vi "TestExec.Example Station Module.vi"(11 "Module Config":T1={"Name"="CircleTest", "Parent Q"=refnum, "Is Child?"=FALSE, "Index"=0, "Dirs"={"Root"=path "", "Config"=path "C:/ATE/Config", "Logs"=path "C:/ATE/Logs", "Reports"=path "C:/ATE/Reports", "App Data"=path "C:/ProgramData/MAIN"}, "Simulate"=FALSE, "SimCtrl"=refnum}) -> ()   [LabVIEW 2018]
uses:
  <vilib>/KATE/Queues/Queue Utils.lvlib
  <vilib>/KATE/Module/Module Utils.lvlib
  <vilib>/KATE/Module/Window/Window.Task, Action.ctl
  <vilib>/KATE/Event Log/Event Log.lvlib
  <vilib>/KATE/Scheduler/Scheduler.lvlib
  <vilib>/KATE/Menu/Menu Utils.lvlib
  <vilib>/KATE/Config/Config Utils.lvlib
  Base Station/Circle Test/Controls & TypeDefs/CircleTest.Config, Track Object Table.ctl
  Common/Utils/Logging/Log Level.ctl
  Common/Utils/Logging/Log Params.ctl
  <vilib>/KATE/Config/Stored Controls/Class.SaveCtrls.lvclass
  <vilib>/KATE/Queues/Q.Element.ctl
  <vilib>/KATE/Module/Module Config.ctl
  <vilib>/KATE/Module/Module.Working Dirs.ctl
  <vilib>/KATE/Module/Module.SW Version Info.ctl
panel:
  in  "Main Tab":enum32{"Operate", "Maint"}(tab)
  out "Simulate Indication":string="Simulating Instruments"
  in  "Data Tab":enum32{"Test Control", "Config"}(tab)
  out "Status":string
  in  "Logging Level":i32
  out "Rev":string="v1.0.0"
  in  "Leave Maint":bool
  in  "SW Rev":T3={"AppName"="Circle Test", "Company"="Valve", "Version"="1.0", "Description"="", "PN"=""}
  # "Title"
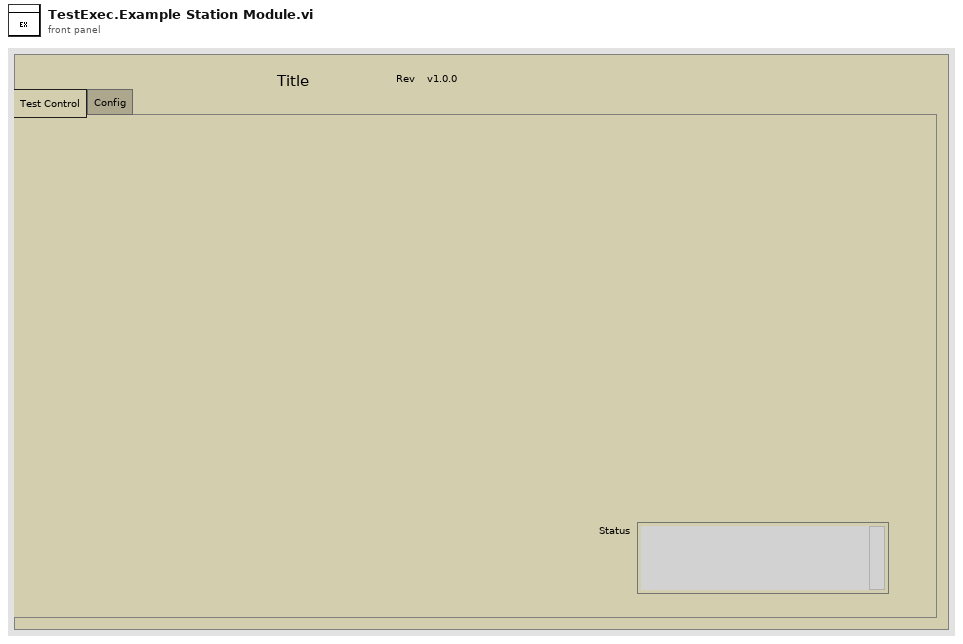
[diagram p1: front panel]
types:
  T1 = typedef "KATE_Lib.lvlib/Module Utils.lvlib/Module Config.ctl" = cluster{"Name":string, "Parent Q":refnum<queue>, "Is Child?":bool, "Index":i32, "Dirs":T2, "Simulate":bool, "SimCtrl":refnum<vi>}
  T2 = typedef "KATE_Lib.lvlib/Module Utils.lvlib/Module.Working Dirs.ctl" = cluster{"Root":path, "Config":path, "Logs":path, "Reports":path, "App Data":path}
  T3 = typedef "KATE_Lib.lvlib/Module Utils.lvlib/Module.SW Version Info.ctl" = cluster{"AppName":string, "Company":string, "Version":string, "Description":string, "PN":string}
  T4 = typedef "KATE_Lib.lvlib/Module Utils.lvlib/Module Sys Info.ctl" = cluster{"Main Q":refnum<queue>, "Exe":bool, "SW Rev":T3, "Self Ref":refnum<vi>, "Main Tab":refnum<vi>, "Pane":refnum<vi>, "Stop":cluster{"Ref":refnum<event-registration>, "Event":refnum<user-event>}, "Cfg":T1, "Services":cluster{"Name":string, "vi ref":refnum<vi>}[], "Menu Ref":refnum<k9>, "CtrlStates":refnum<class "Class.SaveCtrls.lvclass">, "Docs":cluster{"Tags":string[], "Paths":path[]}, "Log":refnum<class "Event Notification.lvclass">, "Test Controls":refnum<vi>[], "Child Modules":cluster{"Name":string, "vi ref":refnum<vi>}[], "SW Items":string[][], "AppData":refnum<class "Class.AppData.lvclass">}
  T5 = enum8{"Enabled", "Disabled", "Disabled and Grayed Out"}
  T6 = typedef "Log Params.ctl" = cluster{"Log Level":T7, "StatusTxtBoxRef":refnum<vi>, "AppID":string, "Is Child?":bool, "Parent Q":refnum<queue>}
  T7 = typedef "Log Level.ctl" = enum16{"Normal", "Verbose", "Debug0", "Debug1", "Debug2"}
  T8 = typedef "CircleTest.Config, Track Object Table.ctl" = cluster{"SNs":string[], "Enable":bool[]}
  T9 = cluster{"Child Modules":cluster{"VI Ref":refnum<vi>, "Name":string}[]}
  T10 = cluster{"Lnch":bool, "Track Obj Config":T8, "Log":T6, "XX":string, "App":cluster{"Child Modules":cluster{"VI Ref":refnum<vi>, "Name":string}[]}}
  T11 = typedef "KATE_Lib.lvlib/Module Utils.lvlib/Window.Task, Action.ctl" = enum16{"Resize()", "Show Panel(Bool)", "Show Scroll Bars(Bool)", "Dock to SubPanel(SubPanel Ref)", "Undock from SubPanel()", "Return to SubPanel()", "Go To Maint Tab()", "Show Maint Tab(Bool)", "Open Block Diagram()"}
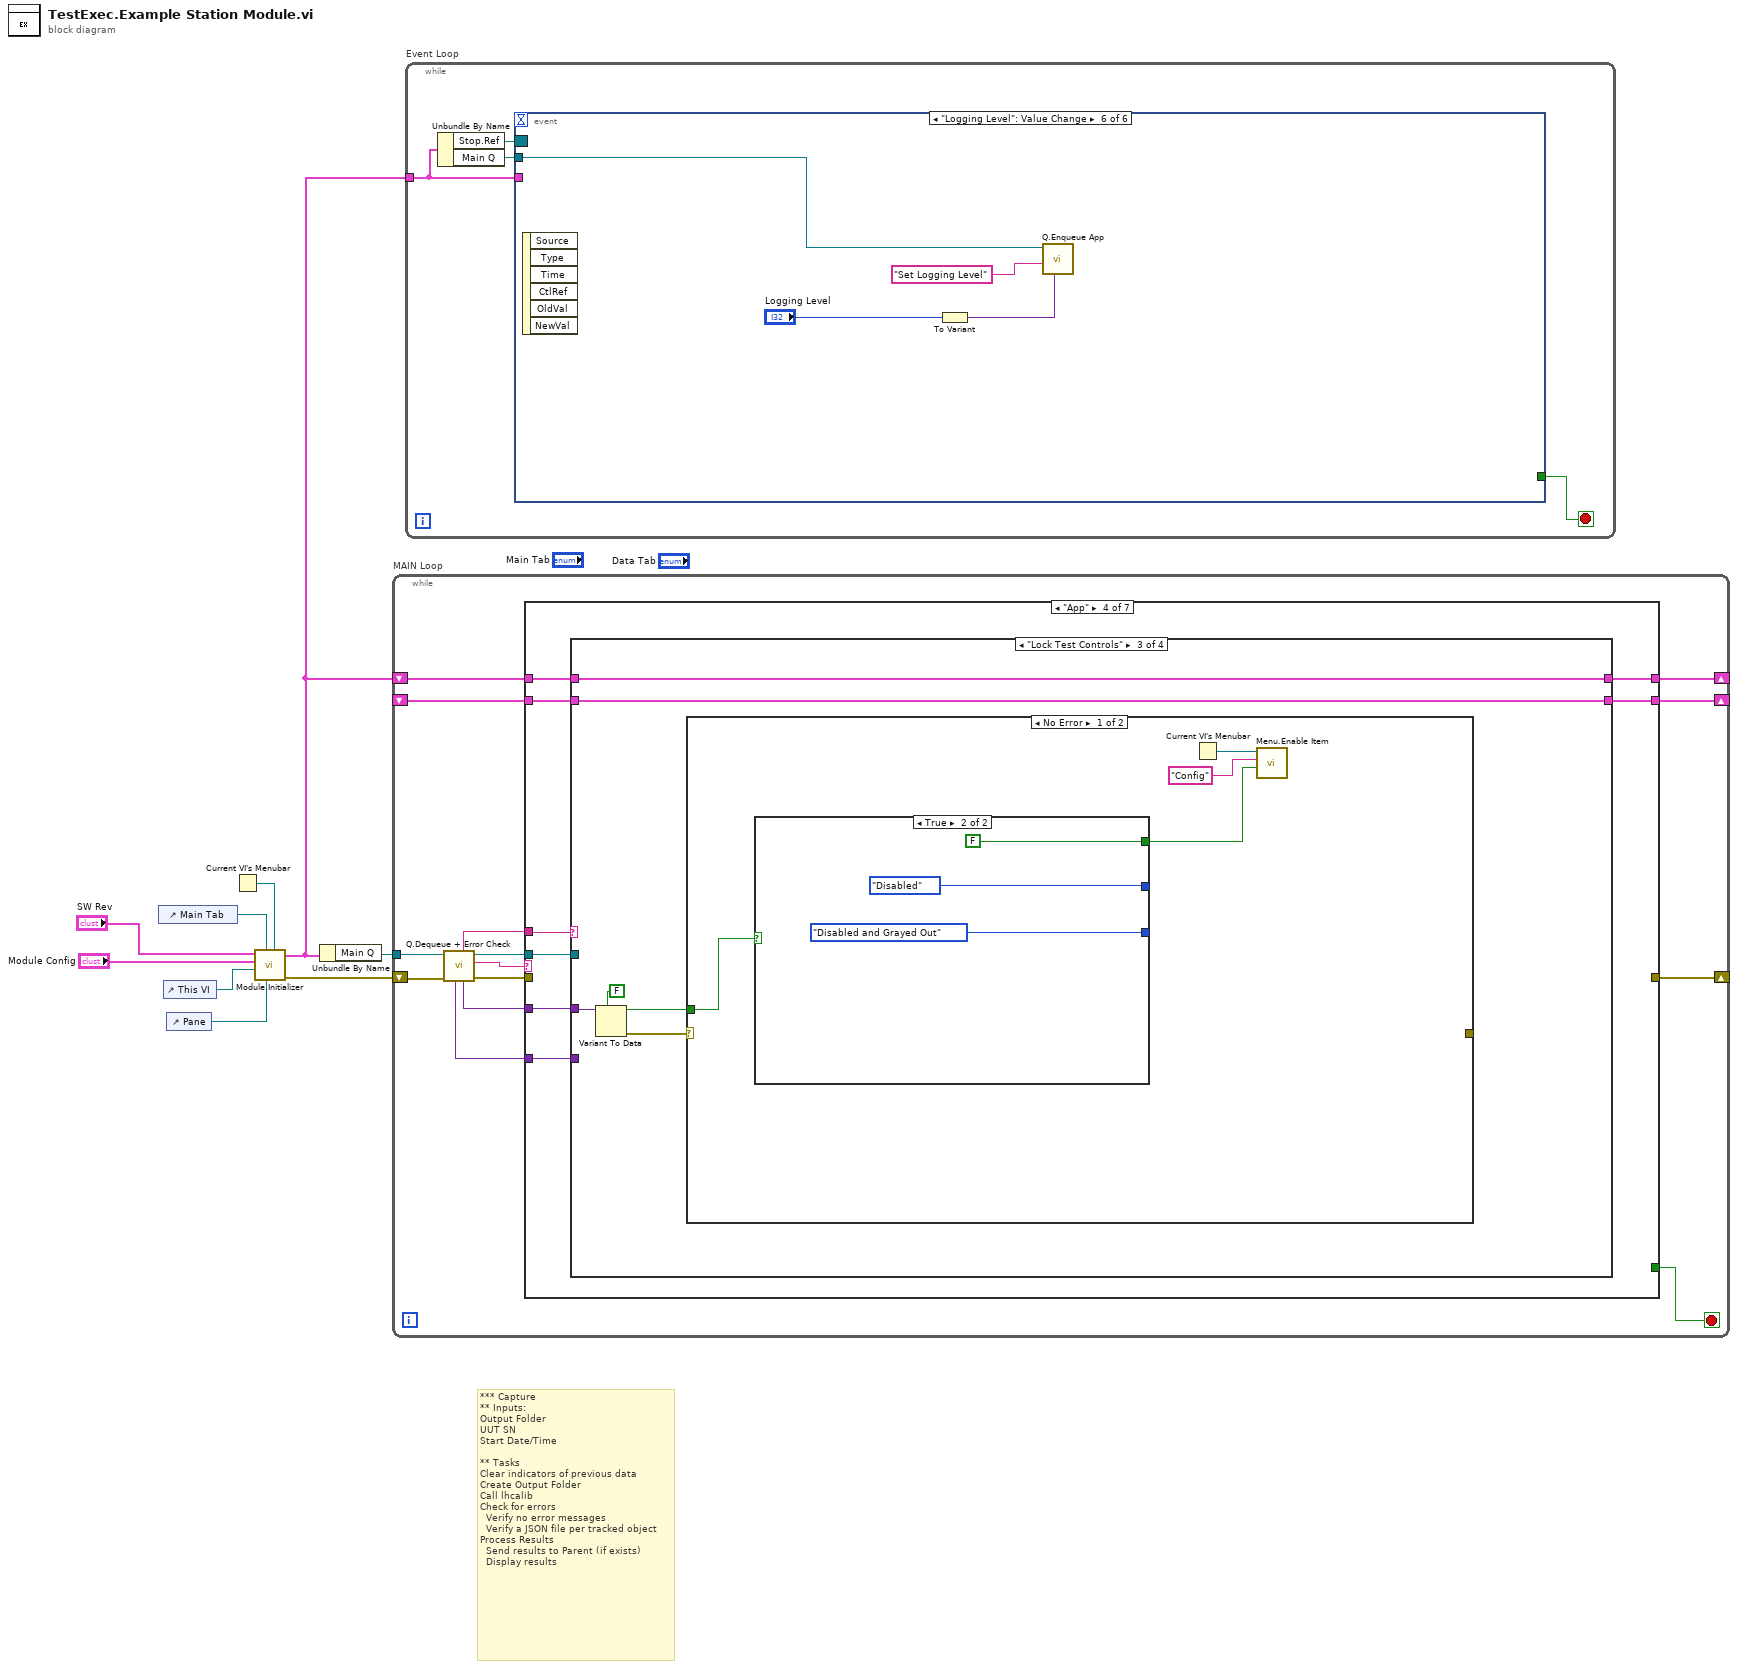
[diagram p0: block diagram]
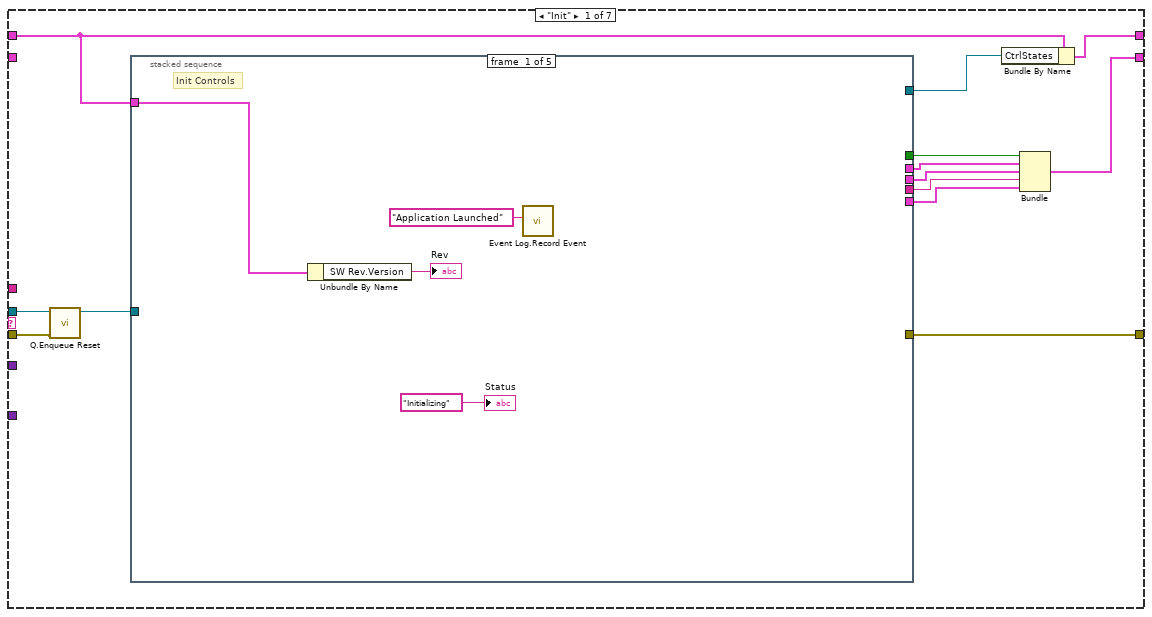
[diagram p2: hidden frame]
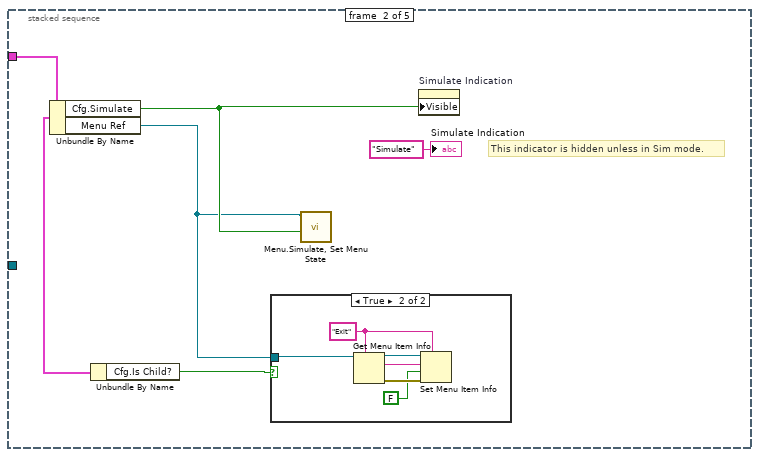
[diagram p3: hidden frame]
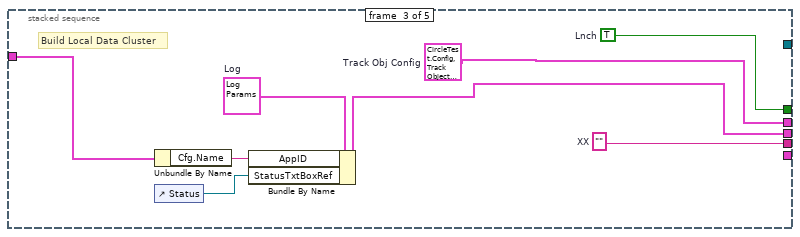
[diagram p5: hidden frame]
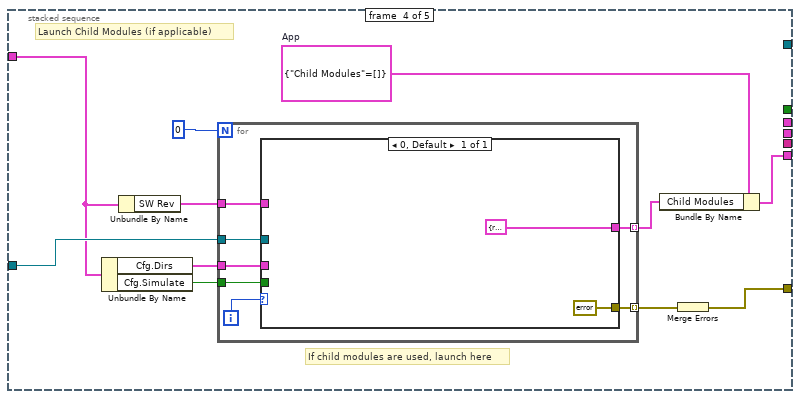
[diagram p6: hidden frame]
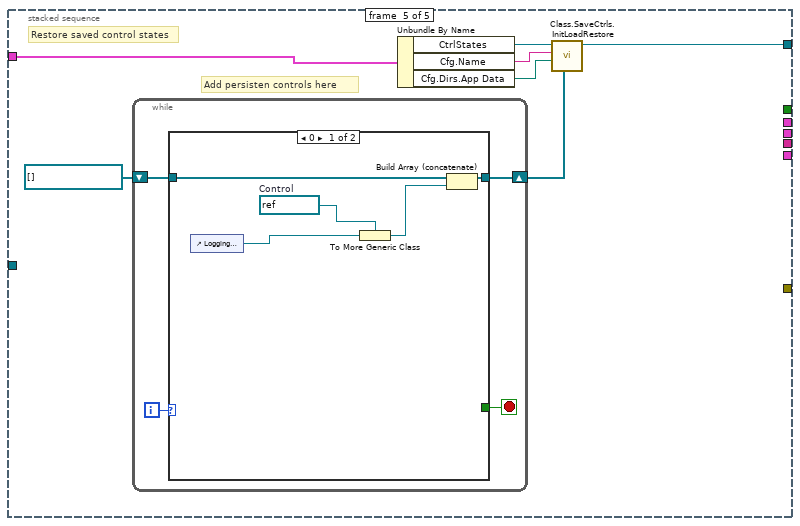
[diagram p7: hidden frame]
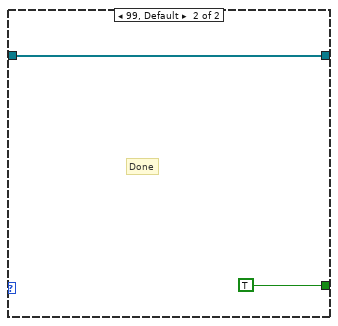
[diagram p8: hidden frame]
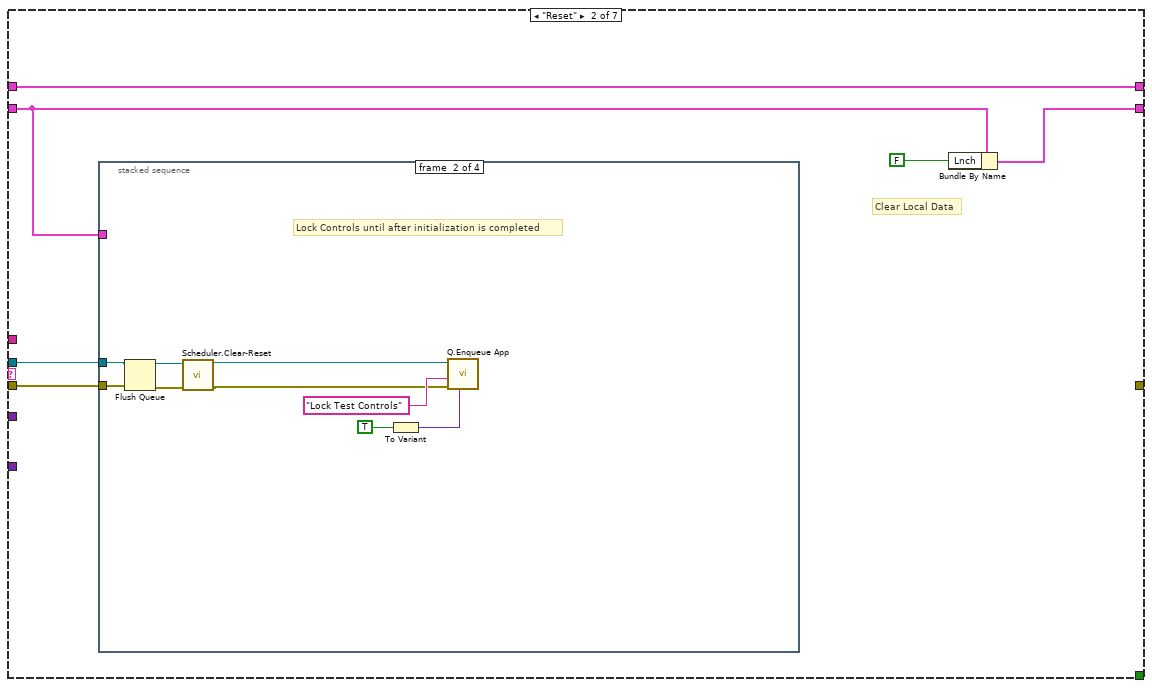
[diagram p9: hidden frame]
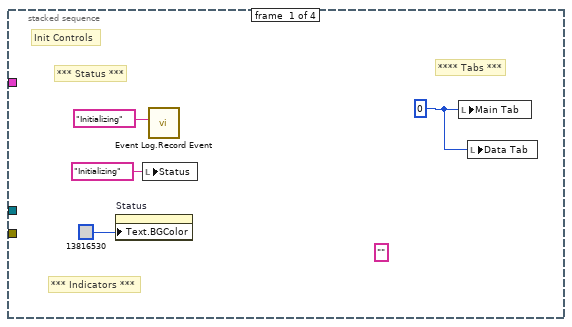
[diagram p10: hidden frame]
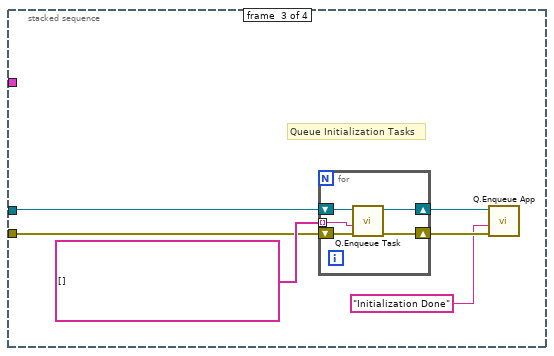
[diagram p11: hidden frame]
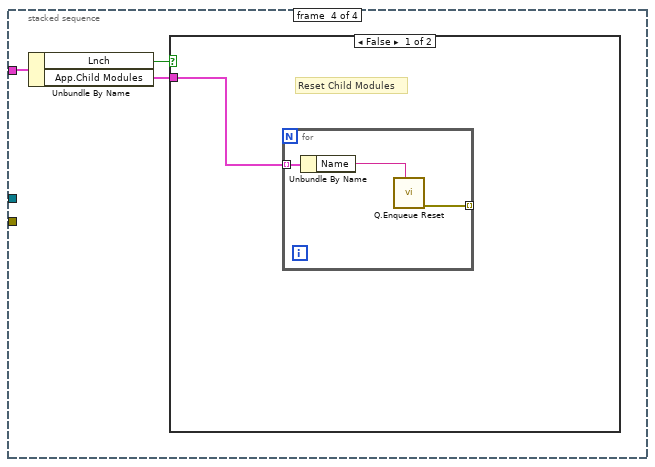
[diagram p12: hidden frame]
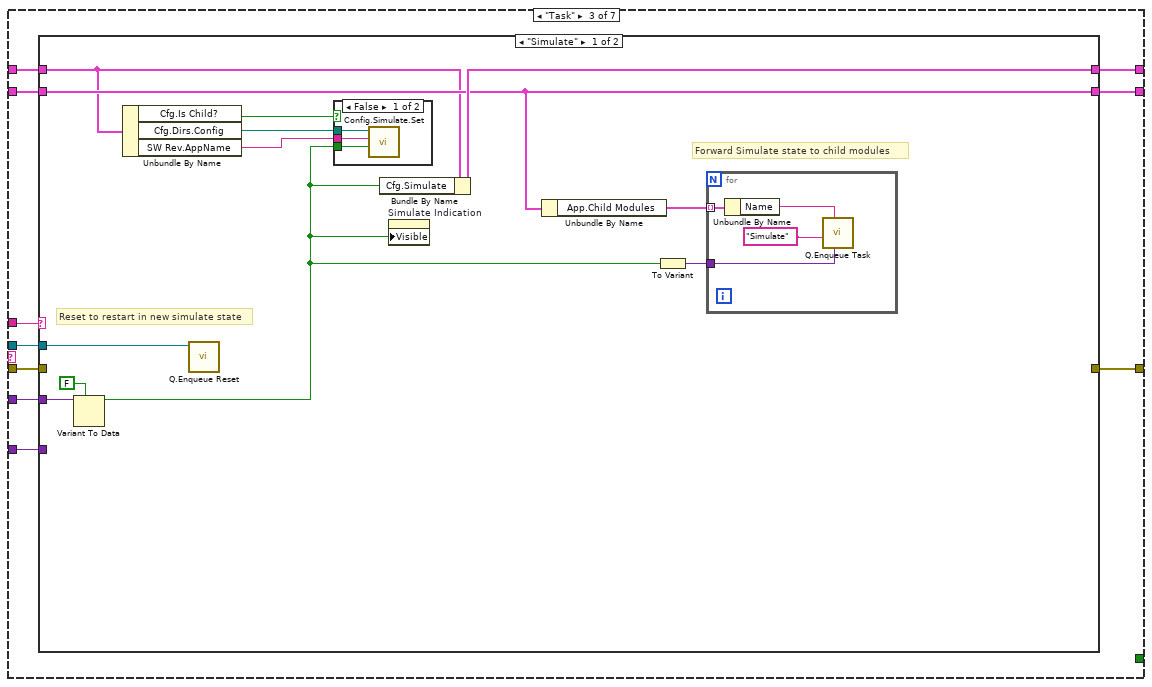
[diagram p14: hidden frame]
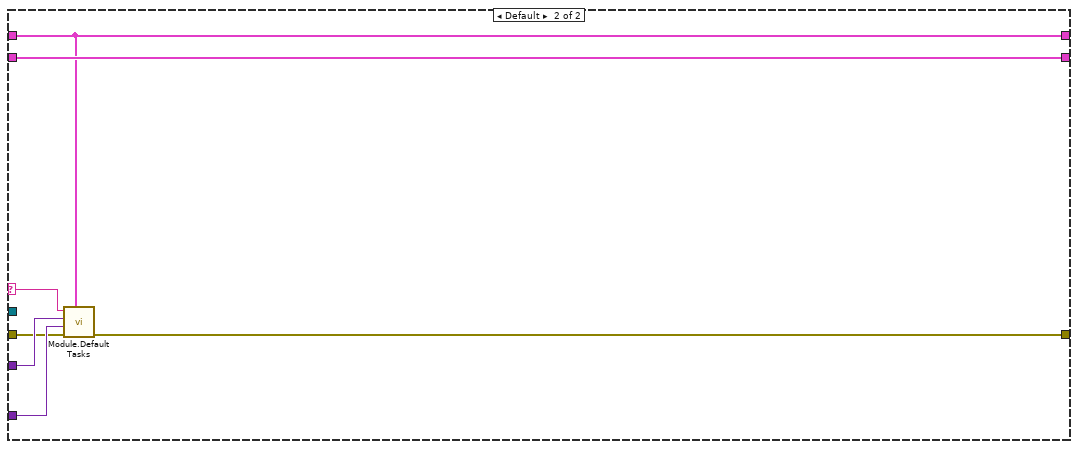
[diagram p16: hidden frame]
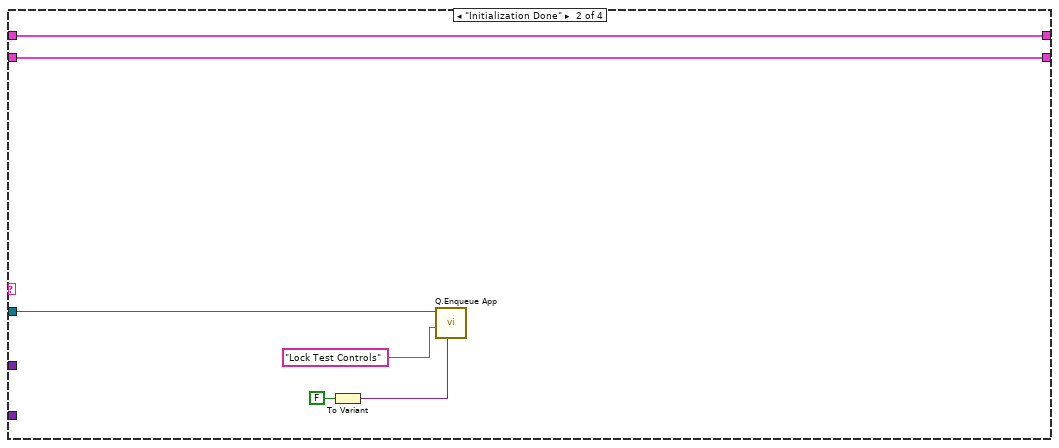
[diagram p18: hidden frame]
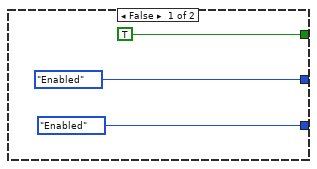
[diagram p19: hidden frame]
diagram:
  # "*** Capture\n** Inputs:\nOutput Folder\nUUT SN\nStart Date/Time\n\n** Tasks \nClear indicators of previous data\nCreate Output Folder\nCall lhcalib\nCheck for errors\n  Verify no error messages\n  Verify a JSON file per tracked object\nProcess Results\n  Send results to Parent (if exists)\n  Display results"
  n1 = control-ref of="Main Tab"() -> (w7:refnum<vi>)
  n2 = control-ref of="This VI"() -> (w6:refnum<vi>)
  n3 = control-ref of="Pane"() -> (w5:refnum<vi>)
  n4 = Current VI's Menubar() -> (w3:refnum<k9>)
  n5 = call <vilib>:"Module.Initializer.vi"("Menu Ref"=w3, "Pane"=w5, "Main Tab"=w7, "Self Ref"=w6, "Module Config"="Module Config", "SW Rev"="SW Rev") -> ("error out"=w9:errorcluster, "Sys"=w4:T4)  [unwired: 4 in]
  n6 = Unbundle By Name(w4) -> ("Main Q"=w8:refnum<queue>)
  n7 = while "MAIN Loop" {
    shift-right: [w19] -> _
    shift-left: w9 -> [w17]
    shift-right: [w20] -> _
    shift-left: _ -> [w23]
    shift-right: [w21] -> _
    shift-left: w4 -> [w22]
    tunnel: w8 -> [w16]
    stop <- w11 stop-if-true
    n8 = call <vilib>:"Q.Dequeue + Error Check.vi"("Error In"=w17, "Q In"=w16) -> ("error out"=w18:errorcluster, "Cmd"=w15:string, "Q Out"=w14:refnum<queue>, "Data1"=w13:variant, "Sub"=w10:string, "Data2"=w12:variant)  [unwired: 4 in]
    n9 = case shown="\"App\"" w15 {
      selector: w15 -> [_ _ _ _ _ w230 _]
      tunnel: w23 -> [_ w99 w143 w173 w220 w232 w259]
      tunnel: w22 -> [w29 w102 w144 w174 w221 w233 w260]
      tunnel: [w30 w102 w142 w172 w219 w233 w260] -> w21
      tunnel: [w34 w103 w141 w171 w218 w232 w259] -> w20
      tunnel: [w26 _ w135 _ w213 w231 w262] -> w19
      tunnel: w18 -> [w35 w100 w137 _ w214 w228 _]
      tunnel: w14 -> [w36 w101 w138 w177 w215 w226 _]
      tunnel: w13 -> [_ _ w139 w176 w216 w229 _]
      tunnel: w12 -> [_ _ w136 w175 w212 _ _]
      tunnel: w10 -> [_ _ w140 w178 w217 w227 _]
      tunnel: [_ _ _ _ _ _ TRUE] -> w11
      frame "Init" {
        n10 = call <vilib>:"Q.Enqueue Reset.vi"("Error In"=w35, "Q In"=w36) -> ("Q Out"=w27:refnum<queue>)  [unwired: 8 in, 1 out]
        n11 = stacked-sequence {
          tunnel: [_ _ w58 _ _] -> w33
          tunnel: [_ _ w56 _ _] -> w32
          tunnel: [_ _ w52 _ _] -> w31
          tunnel: w29 -> [w38 w42 w55 w63 w81]
          tunnel: [_ _ _ _ w80] -> w28
          tunnel: [_ _ _ w69 _] -> w24
          tunnel: w27 -> [_ _ _ w64 _]
          tunnel: [_ _ _ w60 _] -> w26
          tunnel: [_ _ w59 _ _] -> w25
          frame #0 {
            # "Init Controls"
            n12 = Unbundle By Name(w38) -> ("SW Rev.Version"=→"Rev":string)
            n13 = call <vilib>:"Event Log.Record Event.vi"("Message"="Application Launched") -> ()  [unwired: 10 in, 1 out]
            "Status" <- "Initializing" ("Status")
          }
          frame #1 {
            # "This indicator is hidden unless in Sim mode."
            n14 = Unbundle By Name(w42) -> ("Cfg.Simulate"=w44:bool, "Menu Ref"=w41:refnum<k9>)
            n15 = Unbundle By Name(w42) -> ("Cfg.Is Child?"=w43:bool)
            n16 = case shown="True" w43 {
              tunnel: w41 -> [_ w47]
              frame False {
              }
              frame True {
                w49 = "Exit"
                n17 = Get Menu Item Info(7:w49, 11:w47) -> (0:w48:errorcluster, 2:w50:string, 3:w51:refnum<k9>)  [unwired: 1 in, 4 out]
                n18 = Set Menu Item Info(7:w49, 8:w48, 9:FALSE ("enabled"), 10:w50, 11:w51) -> ()  [unwired: 2 in, 2 out]
              }
            }
            n19 = call <vilib>:"Menu.Simulate, Set Menu State.vi"("Sim Enable"=w44, "Menu Ref"=w41) -> ()  [unwired: 8 in, 2 out]
            n20 = property on="Simulate Indication" class="Str"("Visible"=w44) -> ()  [unwired: 2 in, 2 out]
            "Simulate Indication" <- "Simulate" ("Simulate Indication")
          }
          frame #2 {
            w52 = ""  # XX
            w57 = T6 {"Log Level"=enum."Normal", "StatusTxtBoxRef"=refnum, "AppID"="", "Is Child?"=FALSE, "Parent Q"=refnum}  # Log
            w58 = T8 {"SNs"=["", "", "", "", "", "", "", "", "", "", "", "", "", ""], "Enable"=[TRUE, TRUE, TRUE, TRUE, TRUE, TRUE, TRUE, TRUE, TRUE, TRUE, TRUE, TRUE, TRUE, TRUE]}  # Track Obj Config
            w59 = TRUE  # Lnch
            # "Build Local Data Cluster"
            n21 = Unbundle By Name(w55) -> ("Cfg.Name"=w54:string)
            n22 = control-ref of="Status"() -> (w53:refnum<vi>)
            n23 = Bundle By Name(cluster=w57, "AppID"=w54, "StatusTxtBoxRef"=w53) -> (w56:T6)
          }
          frame #3 {
            w70 = T9 {"Child Modules"=[]}  # App
            # "If child modules are used, launch here"
            # "Launch Child Modules (if applicable)"
            n24 = Unbundle By Name(w63) -> ("Cfg.Dirs"=w66:T2, "Cfg.Simulate"=w65:bool)
            n25 = Unbundle By Name(w63) -> ("SW Rev"=w68:T3)
            n26 = for {
              N: 0 -> [_]
              tunnel: w68 -> [w77]
              tunnel: [w72] -> w62 mode=indexing
              tunnel: w64 -> [w75]
              tunnel: w66 -> [w74]
              tunnel: w65 -> [w73]
              tunnel: [w71] -> w61 mode=indexing
              i -> [w76]
              n27 = case shown="0, Default" w76 {
                tunnel: w77 -> [_]
                tunnel: w75 -> [_]
                tunnel: w74 -> [_]
                tunnel: w73 -> [_]
                tunnel: [cluster{"VI Ref":refnum<vi>, "Name":string} {"VI Ref"=refnum, "Name"=""} ("output cluster")] -> w72
                tunnel: [errorcluster {"status"=FALSE, "code"=0, "source"=""} ("error constant")] -> w71
                frame 0, Default {
                }
              }
            }
            n28 = Bundle By Name(cluster=w70, "Child Modules"=w62) -> (w69:T9)
            n29 = Merge Errors(w61) -> (w60:errorcluster)
          }
          frame #4 {
            # "Add persisten controls here"
            # "Restore saved control states"
            n30 = while {
              shift-right: [w88] -> w82
              shift-left: refnum<vi>[] [] -> [w89]
              i -> [w90]
              stop <- w87 stop-if-true
              n31 = case shown="0" w90 {
                tunnel: w89 -> [w94 w97]
                tunnel: [w95 w97] -> w88
                tunnel: [_ TRUE] -> w87
                frame 0 {
                  w92 = refnum<vi> refnum  # Control
                  n32 = control-ref of="Logging Level"() -> (w91:refnum<vi>)
                  n33 = To More Generic Class(target class=w92, reference=w91) -> (generic class reference=w93:refnum<vi>)
                  n34 = Build Array (concatenate)(w94, w93) -> (w95:refnum<vi>[])
                }
                frame 99, Default {
                  # "Done"
                }
              }
            }
            n35 = Unbundle By Name(w81) -> ("CtrlStates"=w83:refnum<class "Class.SaveCtrls.lvclass">, "Cfg.Name"=w85:string, "Cfg.Dirs.App Data"=w84:path)
            n36 = call-dynamic "Class.SaveCtrls.InitLoadRestore.vi"("Ctrl Array"=w82, "Module Data Dir"=w84, "Module Name"=w85, "CtrlStates In"=w83) -> ("CtrlStates"=w80:refnum<class "Class.SaveCtrls.lvclass">)  [unwired: 6 in, 1 out]
          }
        }
        n37 = Bundle By Name(cluster=w29, "CtrlStates"=w28) -> (w30:T4)
        n38 = Bundle("Lnch"=w25, "Track Obj Config"=w33, "Log"=w32, "XX"=w31, "App"=w24) -> (w34:T10)  [unwired: 1 in]
      }
      frame "Reset" {
        # "Clear Local Data"
        n39 = stacked-sequence {
          tunnel: w101 -> [_ w109 w117 _]
          tunnel: w100 -> [_ w108 w121 _]
          tunnel: w99 -> [_ _ _ w130]
          frame #0 {
            (unwired) "" ("Log")
            w104 = 0
            # "*** Indicators ***"
            # "**** Tabs ***"
            # "*** Status ***"
            # "Init Controls"
            n40 = property on="Status" class="Str"("Text.BGColor"=u32 13816530) -> ()  [unwired: 2 in, 2 out]
            n41 = local write "Status"("Initializing" ("Status")) -> ()
            n42 = call <vilib>:"Event Log.Record Event.vi"("Message"="Initializing") -> ()  [unwired: 10 in, 1 out]
            n43 = local write "Main Tab"(w104) -> ()
            n44 = local write "Data Tab"(w104) -> ()
          }
          frame #1 {
            # "Lock Controls until after initialization is completed"
            n45 = Flush Queue(queue=w109, error in (no error)=w108) -> (queue out=w110:refnum<queue>, error out=w113:errorcluster)  [unwired: 1 out]
            n46 = call <vilib>:"Scheduler.Clear-Reset.vi"("error in"=w113, "Q In"=w110) -> ("error out"=w111:errorcluster, "Q Out"=w112:refnum<queue>)  [unwired: 8 in]
            n47 = To Variant(anything=TRUE) -> (Variant=w115:variant)
            n48 = call <vilib>:"Q.Enqueue App.vi"("Data1"=w115, "Error In"=w111, "Task Name"="Lock Test Controls", "Q In"=w112) -> ()  [unwired: 6 in, 2 out]
          }
          frame #2 {
            # "Queue Initialization Tasks"
            n49 = for {
              shift-right: [w125] -> w119
              shift-left: w121 -> [w126]
              tunnel: string[] [] -> [w123] mode=indexing
              shift-right: [w124] -> w120
              shift-left: w117 -> [w127]
              n50 = call <vilib>:"Q.Enqueue Task.vi"("Error In"=w126, "Task Name"=w123, "Q In"=w127) -> ("error out"=w125:errorcluster, "Q Out"=w124:refnum<queue>)  [unwired: 7 in]
            }
            n51 = call <vilib>:"Q.Enqueue App.vi"("Error In"=w119, "Task Name"="Initialization Done", "Q In"=w120) -> ()  [unwired: 7 in, 2 out]
          }
          frame #3 {
            n52 = Unbundle By Name(w130) -> ("Lnch"=w129:bool, "App.Child Modules"=w128:cluster{"VI Ref":refnum<vi>, "Name":string}[])
            n53 = case shown="False" w129 {
              tunnel: w128 -> [w131 _]
              frame False {
                # "Reset Child Modules"
                n54 = for {
                  tunnel: w131 -> [w134] mode=indexing
                  tunnel: [w132] -> _ mode=indexing
                  n55 = Unbundle By Name(w134) -> ("Name"=w133:string)
                  n56 = call <vilib>:"Q.Enqueue Reset.vi"("Q Name"=w133) -> ("error out"=w132:errorcluster)  [unwired: 9 in, 1 out]
                }
              }
              frame True {
                # "Do not reset at launch.\nThey are already reset"
              }
            }
          }
        }
        n57 = Bundle By Name(cluster=w99, "Lnch"=FALSE ("Test.Running")) -> (w103:T10)
      }
      frame "Task" {
        n58 = case shown="\"Simulate\"" w140 {
          selector: w140 -> [_ w168]
          tunnel: w144 -> [w149 w169]
          tunnel: w143 -> [w153 w170]
          tunnel: [w154 w169] -> w142
          tunnel: [w153 w170] -> w141
          tunnel: w139 -> [w156 w167]
          tunnel: w138 -> [w150 _]
          tunnel: w137 -> [_ w165]
          tunnel: w136 -> [_ w166]
          tunnel: [_ w164] -> w135
          frame "Simulate" {
            # "Reset to restart in new simulate state"
            # "Forward Simulate state to child modules"
            n59 = Variant To Data(type=FALSE, Variant=w156) -> (data=w146:bool)  [unwired: 1 in, 1 out]
            n60 = Unbundle By Name(w149) -> ("Cfg.Is Child?"=w145:bool, "Cfg.Dirs.Config"=w148:path, "SW Rev.AppName"=w147:string)
            n61 = call <vilib>:"Q.Enqueue Reset.vi"("Q In"=w150) -> ()  [unwired: 9 in, 2 out]
            n62 = case shown="False" w145 {
              tunnel: w148 -> [w159 _]
              tunnel: w147 -> [w158 _]
              tunnel: w146 -> [w157 _]
              frame False {
                n63 = call <vilib>:"Config.Simulate.Set.vi"("Simulate"=w157, 10:w158, "Config Folder"=w159) -> ()  [unwired: 8 in, 1 out]
              }
              frame True {
              }
            }
            n64 = Bundle By Name(cluster=w149, "Cfg.Simulate"=w146) -> (w154:T4)
            n65 = property on="Simulate Indication" class="Str"("Visible"=w146) -> ()  [unwired: 2 in, 2 out]
            n66 = Unbundle By Name(w153) -> ("App.Child Modules"=w152:cluster{"VI Ref":refnum<vi>, "Name":string}[])
            n67 = To Variant(anything=w146) -> (Variant=w151:variant)
            n68 = for {
              tunnel: w152 -> [w163] mode=indexing
              tunnel: w151 -> [w160]
              n69 = Unbundle By Name(w163) -> ("Name"=w162:string)
              n70 = call <vilib>:"Q.Enqueue Task.vi"("Data1"=w160, "Q Name"=w162, "Task Name"="Simulate") -> ()  [unwired: 7 in, 2 out]
            }
          }
          frame Default {
            n71 = call <vilib>:"Module.Default Tasks.vi"("Sys"=w169, "error in"=w165, "Data2"=w166, "Data1"=w167, "Sub"=w168) -> ("error out"=w164:errorcluster)  [unwired: 5 in, 1 out]
          }
        }
      }
      frame "App" {
        n72 = case shown="\"Lock Test Controls\"" w178 {
          tunnel: w177 -> [_ w181 _ _]
          tunnel: w176 -> [_ _ w187 w206]
          tunnel: w175 -> [_ _ _ _]
          tunnel: w174 -> [w180 w186 w192 w209]
          tunnel: w173 -> [w179 w185 w191 w208]
          tunnel: [w180 w186 w192 w209] -> w172
          tunnel: [w179 w185 w191 w207] -> w171
          frame Default {
          }
          frame "Initialization Done" {
            n73 = To Variant(anything=FALSE) -> (Variant=w183:variant)
            n74 = call <vilib>:"Q.Enqueue App.vi"("Data1"=w183, "Task Name"="Lock Test Controls", "Q In"=w181) -> ()  [unwired: 7 in, 2 out]
          }
          frame "Lock Test Controls" {
            n75 = Variant To Data(type=FALSE, Variant=w187) -> (data=w188:bool, error out=w189:errorcluster)  [unwired: 1 in]
            n76 = case shown="No Error" w189 {
              selector: w189 -> [_ w203]
              tunnel: w188 -> [w196 _]
              tunnel: [_ w203] -> _
              frame No Error {
                n77 = case shown="True" w196 {
                  tunnel: [T5."Enabled" ("Disabled") T5."Disabled and Grayed Out" ("Disabled")] -> _
                  tunnel: [T5."Enabled" ("Disabled") T5."Disabled" ("Disabled")] -> _
                  tunnel: [TRUE ("Enable") FALSE ("Enable")] -> w193
                  frame False {
                  }
                  frame True {
                  }
                }
                n78 = Current VI's Menubar() -> (w194:refnum<k9>)
                n79 = call <vilib>:"Menu.Enable Item.vi"("Enable"=w193, "Tag"="Config", "Menu Ref"=w194) -> ()  [unwired: 7 in, 2 out]
              }
              frame Error {
              }
            }
          }
          frame "Set Logging Level" {
            n80 = Variant To Data(type=0, Variant=w206) -> (data=w204:i32)  [unwired: 1 in, 1 out]
            n81 = Bundle By Name(cluster=w208, "Log.Log Level"=w204) -> (w207:T10)
          }
        }
      }
      frame "Function" {
        n82 = case shown="Default" w217 {
          tunnel: w221 -> [w224]
          tunnel: w220 -> [w225]
          tunnel: [w224] -> w219
          tunnel: [w225] -> w218
          tunnel: w216 -> [_]
          tunnel: w215 -> [_]
          tunnel: w214 -> [w222]
          tunnel: w212 -> [_]
          tunnel: [w222] -> w211
          tunnel: [variant] -> w210
          frame Default {
            # "Do nothing.  The sender of the command will report an error (timeout or incorrect data)."
          }
        }
        n83 = call <vilib>:"Q.Return Function Data.vi"("error in"=w211, "Data2"=w212, "Ret Data"=w210) -> ("error out"=w213:errorcluster)  [unwired: 8 in]
      }
      frame "Error", Default {
        n84 = case shown="\"Error\"" w230 {
          selector: w230 -> [_ w252]
          tunnel: [w235 w253] -> w231
          tunnel: w229 -> [w241 _]
          tunnel: w228 -> [w239 _]
          tunnel: w227 -> [w240 _]
          tunnel: w226 -> [w237 _]
          frame "Error" {
            n85 = case shown="\"Error\"" w240 {
              tunnel: w241 -> [_ w251]
              tunnel: w239 -> [w247 _]
              tunnel: [w247 w249] -> w234
              tunnel: w237 -> [w246 w248]
              tunnel: [w246 w248] -> w236
              frame Default {
              }
              frame "Error" {
                n86 = Variant To Data(type=errorcluster {"status"=FALSE, "code"=0, "source"=""} ("error constant"), Variant=w251) -> (data=w249:errorcluster)  [unwired: 1 in, 1 out]
              }
            }
            n87 = call "Dialog.Error Message.vi"("error in"=w234) -> ("Selection"=w238:enum16{"Exit", "Reset", "Ignore"})
            n88 = call <vilib>:"Event Log.Record Event.vi"("error in"=w234) -> ()  [unwired: 10 in, 1 out]
            n89 = case shown="\"Reset\"" w238 {
              tunnel: w236 -> [w243 _ w245]
              tunnel: [w242 _ w244] -> w235
              frame "Exit", Default {
                n90 = call <vilib>:"Q.Enqueue Exit.vi"("Q In"=w243) -> ("error out"=w242:errorcluster)  [unwired: 9 in, 1 out]
              }
              frame "Ignore" {
              }
              frame "Reset" {
                n91 = call <vilib>:"Q.Enqueue Reset.vi"("Q In"=w245) -> ("error out"=w244:errorcluster)  [unwired: 9 in, 1 out]
              }
            }
          }
          frame Default {
            n92 = Concatenate Strings("Undefined State: \"", w252, "\".") -> (w254:string)
            n93 = Bundle By Name(cluster=errorcluster {"status"=TRUE, "code"=-5000, "source"=""} ("error constant"), "source"=w254) -> (w253:errorcluster)
          }
        }
      }
      frame "Exit" {
        # "This connection is made to not close\n the module until exit tasks are done."
        n94 = stacked-sequence {
          tunnel: w259 -> [_ w264]
          tunnel: [errorcluster {"status"=FALSE, "code"=0, "source"=""} ("error constant") _] -> w258
          frame #0 {
            # "Close connection to instruments"
          }
          frame #1 {
            # "Leave error not connected\nIgnore errors"
            # "Send Exit command to child modules"
            n95 = Unbundle By Name(w264) -> ("App.Child Modules"=w265:cluster{"VI Ref":refnum<vi>, "Name":string}[])
            n96 = for {
              tunnel: w265 -> [w268] mode=indexing
              tunnel: [w266] -> _ mode=indexing
              n97 = Unbundle By Name(w268) -> ("Name"=w267:string)
              n98 = call <vilib>:"Q.Enqueue Exit.vi"("Q Name"=w267) -> ("error out"=w266:errorcluster)  [unwired: 9 in, 1 out]
            }
          }
        }
        n99 = call <vilib>:"Module.Destructor.vi"("error in"=w258, "Sys"=w260) -> ("error out"=w262:errorcluster)  [unwired: 9 in]
      }
    }
  }
  n100 = while "Event Loop" {
    tunnel: w4 -> [w271]
    stop <- w272 stop-if-true
    n101 = Unbundle By Name(w271) -> ("Stop.Ref"=w270:refnum<event-registration>, "Main Q"=w269:refnum<queue>)
    n102 = event shown="[5] \"Logging Level\": Value Change" {
      selector: w270 -> [_ _ _ _ _ _]
      dyn-events: _ -> [_ _ _ _ _ _]
      timeout: _ -> [_ _ _ _ _ _]
      tunnel: [w275 _ _ w293 TRUE _] -> w272
      tunnel: w271 -> [w274 _ _ w291 _ _]
      tunnel: w269 -> [w277 w287 _ w292 _ w317]
      event Panel Close? {
        n103 = event-data() -> ()  [unwired: 1 in, 4 out]
        n104 = Unbundle By Name(w274) -> ("Cfg.Is Child?"=w273:bool)
        n105 = case shown="True" w273 {
          tunnel: w277 -> [w280 w283]
          tunnel: [TRUE TRUE] -> w276
          tunnel: [TRUE FALSE] -> w275
          tunnel: [_ w281] -> _
          frame False {
            # "Parent - Exit"
            n106 = call <vilib>:"Q.Enqueue Exit.vi"("Q In"=w280) -> ()  [unwired: 9 in, 2 out]
          }
          frame True {
            # "Child - Hide Panel and if was \nin a subpanel, return to subpanel."
            n107 = call <vilib>:"Module.Window, Q Task.vi"("Action"=Window.Task,_Action."Return to SubPanel()", "Q In"=w283) -> ("error out"=w281:errorcluster)  [unwired: 8 in, 1 out]
          }
        }
        n108 = event-data("Discard?"=w276) -> ()  [unwired: 1 in, 1 out]
      }
      event Panel Resize {
        n109 = event-data() -> ()  [unwired: 1 in, 8 out]
        n110 = call <vilib>:"Module.Window, Q Task.vi"("Action"=Window.Task,_Action."Resize()", "Q In"=w287) -> ()  [unwired: 8 in, 2 out]
      }
      event "Leave Maint": Value Change {
        n111 = event-data() -> ()  [unwired: 1 in, 6 out]
        n112 = local write "Main Tab"(0) -> ()
      }
      event Menu Selection (User) {
        n113 = event-data() -> ("MenuRef"=w289:refnum<k9>, "ItemTag"=w290:string)  [unwired: 1 in, 5 out]
        n114 = case shown="\"Help.About\"" w290 {
          selector: w290 -> [w295 _ _ _ _ w305 _ _]
          tunnel: [_ TRUE _ _ _ _ _ _] -> w293
          tunnel: w292 -> [_ w298 _ w301 _ w309 w311 w313]
          tunnel: [_ _ w300 _ _ _ _ _] -> _
          tunnel: w291 -> [w294 _ _ _ w303 _ _ _]
          tunnel: w289 -> [_ _ _ _ _ w306 _ _]
          frame Default {
            # "Check if a help document was selected.\nIf so, open the document"
            n115 = Unbundle By Name(w294) -> ("Docs.Tags"=w297:string[], "Docs.Paths"=w296:path[])
            n116 = call <vilib>:"Menu.Help, Open User Manual Items.vi"("Menu Tag Selection"=w295, "Paths"=w296, "Tags"=w297) -> ()  [unwired: 8 in, 1 out]
          }
          frame "Exit" {
            n117 = call <vilib>:"Q.Enqueue Exit.vi"("Q In"=w298) -> ()  [unwired: 9 in, 2 out]
          }
          frame "Event Log" {
            n118 = call <vilib>:"Event Log.Show.vi"() -> ("error out"=w300:errorcluster)  [unwired: 11 in]
          }
          frame "Reset" {
            n119 = call <vilib>:"Q.Enqueue Reset.vi"("Q In"=w301) -> ()  [unwired: 9 in, 2 out]
          }
          frame "Help.About" {
            n120 = Unbundle By Name(w303) -> ("SW Rev"=w302:T3)
            n121 = call <vilib>:"Help.About.vi"("SW Version"=w302) -> ()  [unwired: 11 in]
          }
          frame "Simulate OFF", "Simulate ON" {
            n122 = call <vilib>:"Menu.Simulate, Set Menu State.vi"("Menu Tag"=w305, "Menu Ref"=w306) -> ("Sim ON"=w304:bool)  [unwired: 8 in, 1 out]
            n123 = To Variant(anything=w304) -> (Variant=w308:variant)
            n124 = call <vilib>:"Q.Enqueue Task.vi"("Data1"=w308, "Task Name"="Simulate", "Q In"=w309) -> ()  [unwired: 7 in, 2 out]
          }
          frame "Show Block Diagram" {
            n125 = call <vilib>:"Module.Window, Q Task.vi"("Action"=Window.Task,_Action."Open Block Diagram()", "Q In"=w311) -> ()  [unwired: 8 in, 2 out]
          }
          frame "Go to Maint Tab" {
            n126 = call <vilib>:"Module.Window, Q Task.vi"("Action"=Window.Task,_Action."Show Maint Tab(Bool)", "Q In"=w313) -> ()  [unwired: 8 in, 2 out]
          }
        }
      }
      event User Event {
        n127 = event-data() -> ()  [unwired: 1 in, 5 out]
      }
      event "Logging Level": Value Change {
        n128 = event-data() -> ()  [unwired: 1 in, 6 out]
        n129 = To Variant(anything="Logging Level") -> (Variant=w315:variant)
        n130 = call <vilib>:"Q.Enqueue App.vi"("Data1"=w315, "Task Name"="Set Logging Level", "Q In"=w317) -> ()  [unwired: 7 in, 2 out]
      }
    }
  }
